vi "INV_step_prompt.vi"(8 "error in":errorcluster, 10 "step":T3={"step_description (prompt)"="", "save results"=FALSE, "step_type"=enum."prompt", "Step_name"="", "bool"=[], "data_unit"=enum."bool", "dbl"=[], "I32"=[], "string"=[]} {"dbl" format="%.3f"}, 11 "Cluster in":T5) -> (0 "error out":errorcluster, 2 "test results":T1, 3 "Cluster out":T5)   [LabVIEW 2020]
uses:
  MPB/controls/test_control.ctl
  MPB/controls/from_PLC.ctl
  MPB/controls/to_PLC.ctl
  controls/Inverter_step.ctl
  controls/Inverter_step_type.ctl
  MPB/controls/data type.ctl
  controls/INV_test results.ctl
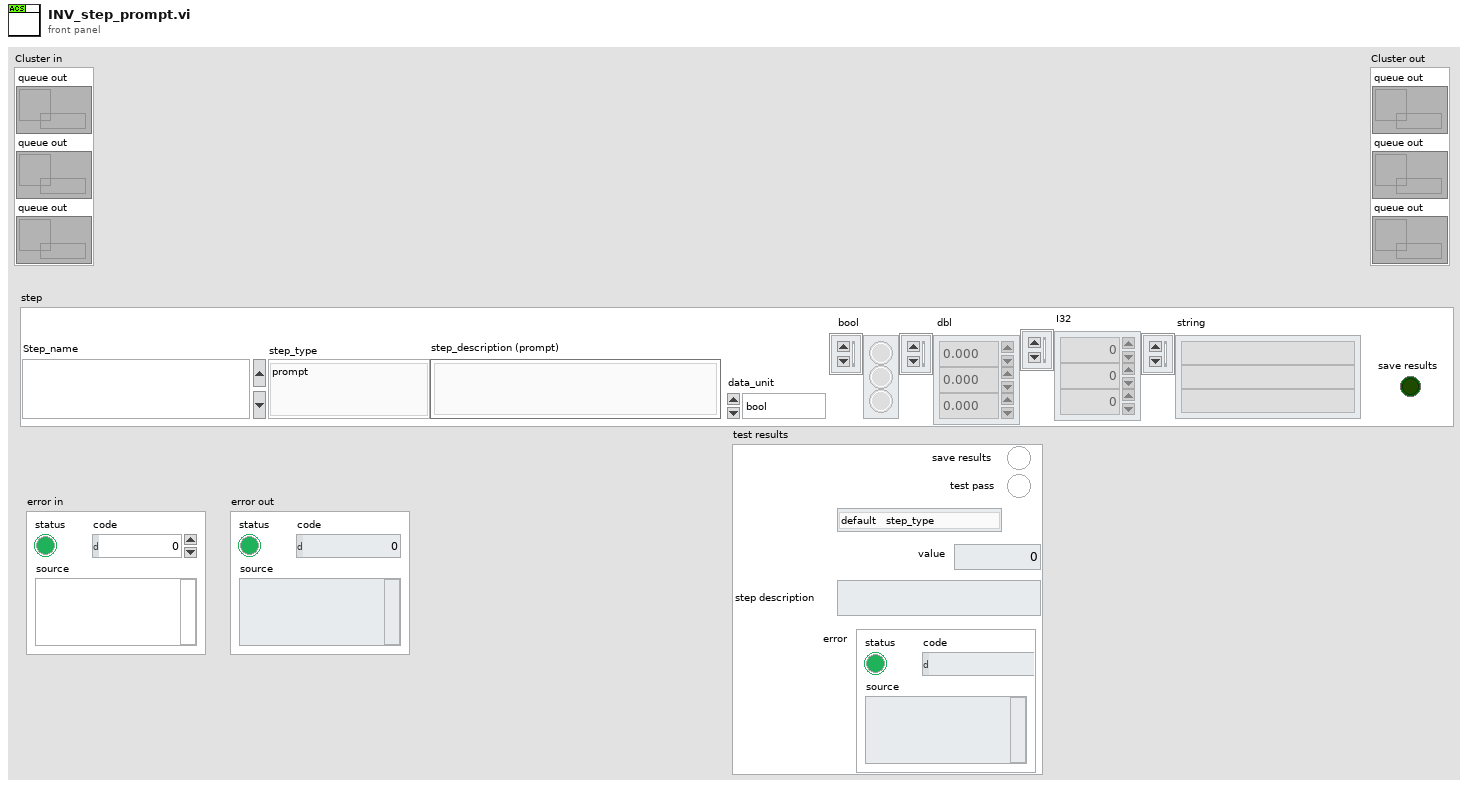
[diagram p1: front panel]
types:
  T1 = typedef "INV_test results.ctl" = cluster{"test pass":bool, "step_type":T2, "value":dbl, "step description":string, "error":errorcluster, "save results":bool}
  T2 = typedef "Inverter_step_type.ctl" = enum16{"default", "prompt", "init_12V_power_supply", "12V_power supply on_off", "write_PLC", "read_PLC", "DAQ_Read", "DAQ_Write", "run .bat file", "display_version", "set flow rate", "init_chroma", "set_chroma_V", "set_chroma_ramp", "wait (sec)", "end_of_test", "record_pass_fail"}
  T3 = typedef "Inverter_step.ctl" = cluster{"step_description (prompt)":string, "save results":bool, "step_type":T2, "Step_name":string, "bool":bool[], "data_unit":T4, "dbl":dbl[], "I32":i32[], "string":string[]}
  T4 = typedef "data type.ctl" = enum16{"bool", "string", "I32", "DBL"}
  T5 = cluster{"queue out":refnum<queue>, "queue out":refnum<queue>, "queue out":refnum<queue>}
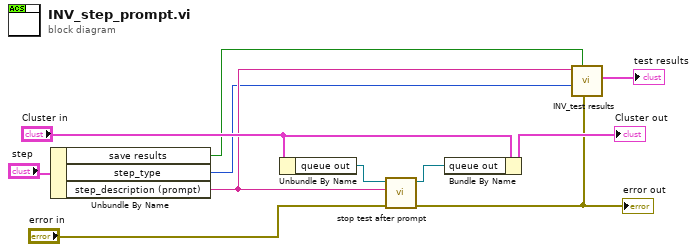
[diagram p0: block diagram]
diagram:
  n1 = Unbundle By Name("step") -> ("save results"=w2:bool, "step_type"=w1:T2, "step_description (prompt)"=w4:string)
  n2 = Unbundle By Name("Cluster in") -> ("queue out"=w10:refnum<queue>)
  n3 = call "stop test after prompt.vi"("error in"="error in", "step_description (prompt)"=w4, "queue in"=w10) -> ("error out"=w3:errorcluster, "queue out"=w11:refnum<queue>)  [unwired: 7 in]
  "error out" <- w3
  n4 = Bundle By Name(cluster="Cluster in", "queue out"=w11) -> (→"Cluster out":T5)
  n5 = call "INV_test results.vi"("error"=w3, "save results"=w2, "step_type"=w1, "(description) used in test"=w4) -> ("test results"=→"test results":T1)  [unwired: 7 in]
